vi "Configure Rx Channel.vi"(8 "error in":errorcluster, 9 "labels settings for RT":T1[](array[typedef]) {"Label Timestamp Channel Data Reference" format="%.0x"; "Word Initial Raw Value" format="%032.0f"; "Label Disable/Trigger Channel Reference" format="%.0x"; "parameter driver data"."Tx parameter refs" format="%.0x"; "SDI" format="%02b"; "label" format="%.0o"}, 10 "channel number in":u8, 11 "board handle in":u8) -> (0 "error out":errorcluster, 2 "channel number out":u8, 3 "board handle out":u8)   [LabVIEW 2024, in "AIM ARINC 429 Hardware API.lvlib"]
doc: "Configures all of the labels for a specified channel to be received."
uses:
  AIM ARINC 429 Hardware API.lvlib
  Shared/RT Label Settings.ctl
  Shared/Label.ctl
  Shared/RT Parameters.ctl
  Shared/Parameter Definition.ctl
  <vilib>/NI/NI VeriStand Encoding and Decoding/Encoding.ctl
  <vilib>/NI VeriStand/Custom Device API/Custom Device Item Ref.ctl
  Shared/Transfer Type.ctl
  <vilib>/NI VeriStand/Custom Device API/Data Reference.ctl
  <instrlib>/AIM GmbH/_ARINC-429/subvi/Error Converter (ErrCode or Status).vi
  <instrlib>/AIM GmbH/_ARINC-429/subvi/Get Library Path.vi
  <instrlib>/AIM GmbH/_ARINC-429/VIs/Library/Api429Lib Error Desc Get.vi
  <instrlib>/AIM GmbH/_ARINC-429/subvi/Get Error Number Offset.vi
  <vilib>/Utility/error.llb/Error Cluster From Error Code.vi
  <instrlib>/AIM GmbH/_ARINC-429/AIM429LV.lvlib
  <vilib>/NI/NI VeriStand Encoding and Decoding/Encoding and Decoding.lvlib
  <vilib>/NI VeriStand/Custom Device API/Custom Device API.lvlib
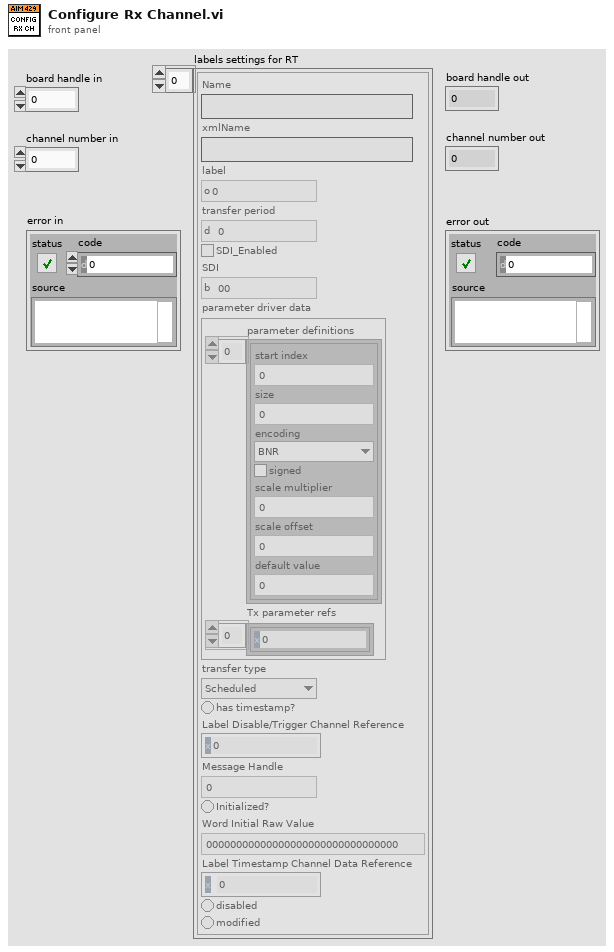
[diagram p1: front panel]
types:
  T1 = typedef "RT Label Settings.ctl" = cluster{"Name":string, "xmlName":string, "label":T2, "transfer period":u32, "SDI_Enabled":bool, "SDI":u8, "parameter driver data":T3, "transfer type":T7, "has timestamp?":bool, "Label Disable/Trigger Channel Reference":T6, "Message Handle":u64, "Initialized?":bool, "Word Initial Raw Value":u32, "Label Timestamp Channel Data Reference":T8, "disabled":bool, "modified":bool}
  T2 = typedef "Label.ctl" = u8
  T3 = typedef "RT Parameters.ctl" = cluster{"parameter definitions":T4[], "Tx parameter refs":T6[]}
  T4 = typedef "Parameter Definition.ctl" = cluster{"start index":i32, "size":i32, "encoding":T5, "signed":bool, "scale multiplier":dbl, "scale offset":dbl, "default value":dbl}
  T5 = typedef "Encoding and Decoding.lvlib/Encoding.ctl" = enum16{"BNR", "BCD", "Discrete"}
  T6 = typedef "Custom Device API.lvlib/Custom Device Item Ref.ctl" = u64
  T7 = typedef "Transfer Type.ctl" = enum16{"Scheduled", "Acyclic", "Block", "Strobe"}
  T8 = typedef "Custom Device API.lvlib/Data Reference.ctl" = i32
  T9 = cluster{"label":u32, "sdi":u32, "con":u32, "irCon":u32, "irIndex":u32, "bufSize":u32}
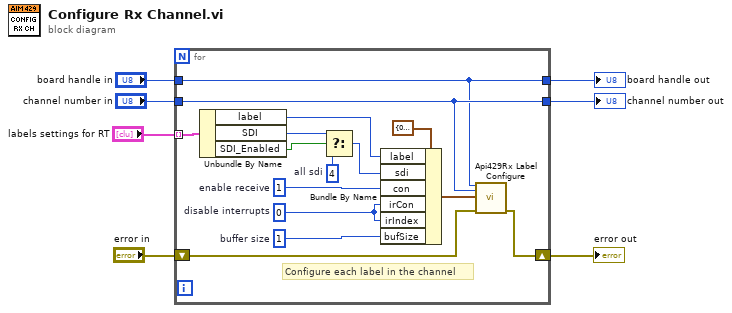
[diagram p0: block diagram]
diagram:
  n1 = for {
    tunnel: "channel number in" -> [w13]
    shift-right: [w21] -> w5
    shift-left: "error in" -> [w22]
    tunnel: "labels settings for RT" -> [w18] mode=indexing
    tunnel: [w13] -> w3
    tunnel: "board handle in" -> [w12]
    tunnel: [w12] -> w1
    w9 = u8 4  # all sdi
    w14 = u32 1  # buffer size
    w15 = u32 0  # disable interrupts
    w16 = u32 1  # enable receive
    # "Configure each label in the channel"
    n2 = Unbundle By Name(w18) -> ("label"=w17:T2, "SDI"=w10:u8, "SDI_Enabled"=w11:bool)
    n3 = Select(t=w10, s=w11, f=w9) -> (s? t:f=w8:u8)
    n4 = Bundle By Name(cluster=T9 {"label"=0, "sdi"=0, "con"=0, "irCon"=0, "irIndex"=0, "bufSize"=0} ("label_setup"), "label"=w17, "sdi"=w8, "con"=w16, "irCon"=w15, "irIndex"=w15, "bufSize"=w14) -> (w20:T9)
    n5 = call <instrlib>:"Api429Rx Label Configure.vi"("board_handle"=w12, "b_Chn"=w13, "label_setup"=w20, "error in (no error)"=w22) -> ("error out"=w21:errorcluster)  [unwired: 9 in, 2 out]
  }
  "board handle out" <- w1
  "channel number out" <- w3
  "error out" <- w5
